vi "Get_User_Name.vi"() -> (0 "User Name":string)   [LabVIEW 2018]
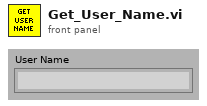
[diagram p1: front panel]
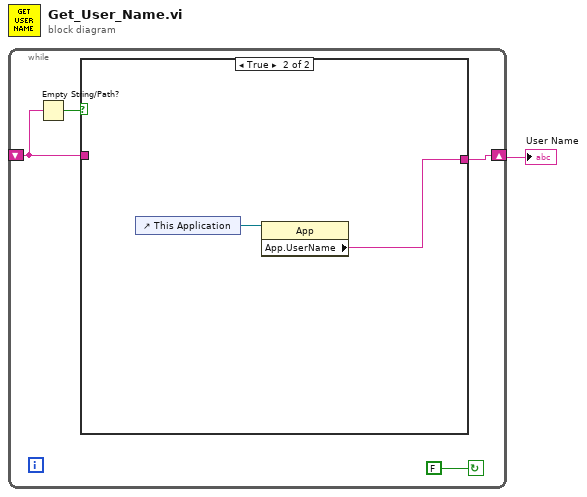
[diagram p0: block diagram]
diagram:
  n1 = while {
    shift-right: [w4] -> w1
    shift-left: _ -> [w2]
    stop <- FALSE continue-if-true
    n2 = Empty String/Path?(string/path=w2) -> (empty?=w3:bool)
    n3 = case shown="True" w3 {
      tunnel: [w6 w7] -> w4
      tunnel: w2 -> [w6 _]
      frame False {
      }
      frame True {
        n4 = control-ref of="This Application"() -> (w8:refnum<vi>)
        n5 = property class="App"(reference=w8) -> ("App.UserName"=w7:string)  [unwired: 1 in, 2 out]
      }
    }
  }
  "User Name" <- w1
